vi "FTW-Supervisor-Connect.vi"(5 "Supervisor Address":string, 11 "error in":errorcluster) -> (4 "FTW Supervisor Connection":refnum<class "FTW-Supervisor-Connector.lvclass">, 15 "error out":errorcluster)   [LabVIEW 2014, in "FTW-Supervisor-Connector.lvclass"]
uses:
  FTW-Supervisor-Connector.lvclass
  FTW-Supervisor-Connector.lvclass/FTW-Supervisor-Connector.ctl
panel:
  # "Inputs"
  # "Outputs"
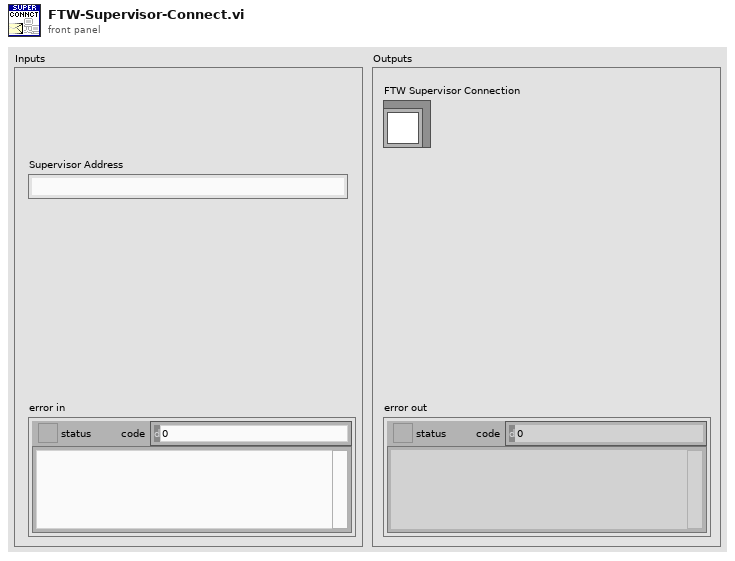
[diagram p1: front panel]
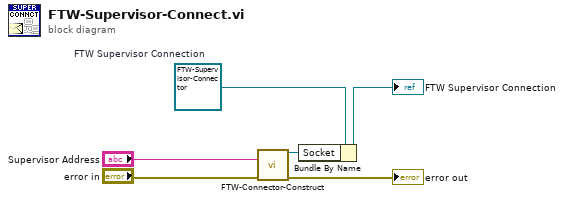
[diagram p0: block diagram]
diagram:
  w3 = refnum<class "FTW-Supervisor-Connector.lvclass"> refnum  # FTW Supervisor Connection
  n1 = call "FTW-Connector-Construct.vi"("Remote Inbox Address"="Supervisor Address", "error in"="error in") -> ("FTW Actor Connector"=w6:refnum<data-value>, "error out"=→"error out":errorcluster)  [unwired: 12 in]
  n2 = Bundle By Name(cluster=w3, "Socket"=w6) -> (→"FTW Supervisor Connection":refnum<class "FTW-Supervisor-Connector.lvclass">)
